vi "DBItemName-Log.vi"() -> (1 "Items":string[](array[string]))   [LabVIEW 2015, in "CopyUtility.lvlib"]
uses:
  CopyUtility.lvlib
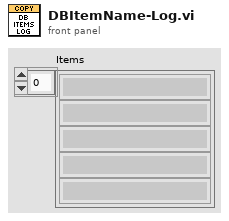
[diagram p1: front panel]
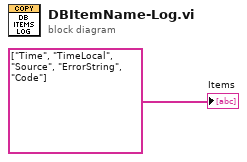
[diagram p0: block diagram]
diagram:
  "Items" <- string[] ["Time", "TimeLocal", "Source", "ErrorString", "Code"]
